vi "Drive Straight.vi"(0 "Distance (ft)":dbl) -> ()   [LabVIEW 2015]
uses:
  <vilib>/Rock Robotics/WPI/Utilities/WPI_GetSetVariantRefNum.vi
  <vilib>/Rock Robotics/WPI/RobotDrive/WPI_RobotDriveArcadeDrive_Standard(NoSaturation).vi
  navX Library v2/navX Library v2.lvlib
panel:
  in  "Ticks/Foot":dbl=442.8
  in  "Drive Straight P":dbl=0.1
  in  "Drive Straight Min":dbl=0.25
  in  "Drive Straight Max":dbl=0.75
  in  "Drive Straight Speed":dbl=0.5 format="%#_13g"
  in  "Drive Straight Tolerance":dbl=1.0
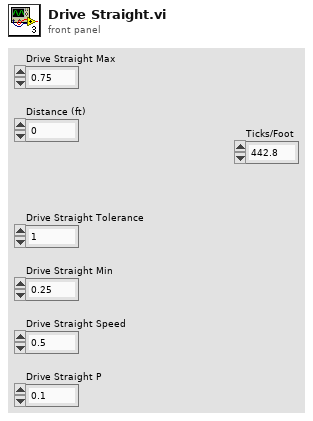
[diagram p1: front panel]
types:
  T1 = typedef "WPI_EncoderDevRef.ctl" = cluster{"DevStatus":errorcluster, "EncoderIndex":T2, "CounterIndex":T3, "DistancePerCount":dbl, "Decoding Type":T4}
  T2 = typedef "FPGA_EncoderIdx.ctl" = enum8{"Enc 0", "Enc 1", "Enc 2", "Enc 3", "Enc 4", "Enc 5", "Enc 6", "Enc 7", "Invalid"}
  T3 = typedef "FPGA_CounterCtrSystemIndex.ctl" = enum8{"Ctr 0", "Ctr 1", "Ctr 2", "Ctr 3", "Ctr 4", "Ctr 5", "Ctr 6", "Ctr 7", "Invalid"}
  T4 = typedef "WPI_EncoderType.ctl" = enum16{"1x", "2x", "4x"}
  T5 = typedef "navX Library v2.lvlib/Z900_navX_DeviceTypeDef.ctl" = cluster{"Interface":cluster{"Protocol":T6, "Update Rate (4Hz-60Hz)":u8, "navX Open TypeDef":variant}, "Notify Packet":refnum<notifier>, "Loop VI Refnum":refnum<vi>, "Ready to Close Occurrence Refnum":refnum<k4>}
  T6 = typedef "navX Library v2.lvlib/Z900_navX_ProtocolTypeDef.ctl" = enum16{"SERIAL", "I2C", "SPI"}
  T7 = cluster{"Yaw":dbl, "Roll":dbl, "Pitch":dbl, "Heading":dbl, "Fused Heading":dbl}
  T8 = typedef "WPI_RobotDriveDevRef.ctl" = cluster{"DevStatus":errorcluster, "Motors[]":T9[], "Square Inputs":bool, "Max Output":dbl}
  T9 = typedef "WPI_MotorControlDeviceRef.ctl" = cluster{"DeviceStatus":errorcluster, "Type":T10, "PWM":cluster{"PWM Channel":T11, "DeadBand":T12}, "CAN":cluster{"Device Number":u8, "Control Mode":T13, "Semaphore":T14, "Max Vout":dbl, "TalonSRX Control Mode":T15}, "Invert":bool}
  T10 = typedef "WPI_MotorControlType.ctl" = enum16{"PWM", "CAN", "CANTalonSRX"}
  T11 = typedef "FPGA_DIOPWMChannel.ctl" = enum8{"PWM 0", "PWM 1", "PWM 2", "PWM 3", "PWM 4", "PWM 5", "PWM 6", "PWM 7", "PWM 8", "PWM 9", "PWM MXP 0", "PWM MXP 1", "PWM MXP 2", "PWM MXP 3", "PWM MXP 4", "PWM MXP 5", "PWM MXP 6", "PWM MXP 7", "PWM MXP 8", "PWM MXP 9", "Invalid"}
  T12 = typedef "WPI_PWMDeadband.ctl" = cluster{"Name":string, "maxPositivePwm":i32, "minPositivePwm":i32, "centerPwm":i32, "maxNegativePwm":i32, "minNegativePwm":i32, "angularRange":u16}
  T13 = typedef "WPI_CANJaguar_ControlMode.ctl" = enum8{"Percent VBus", "Current", "Speed", "Position", "Voltage"}
  T14 = typedef "Semaphore RefNum" = refnum<k1>
  T15 = typedef "WPI_CANTalonSRX_APIControlMode.ctl" = enum8{"Percent VBus", "Speed", "Position", "Slave", "Unchanged / Invalid", "Voltage Compensation", "Current", "Motion Profile"}
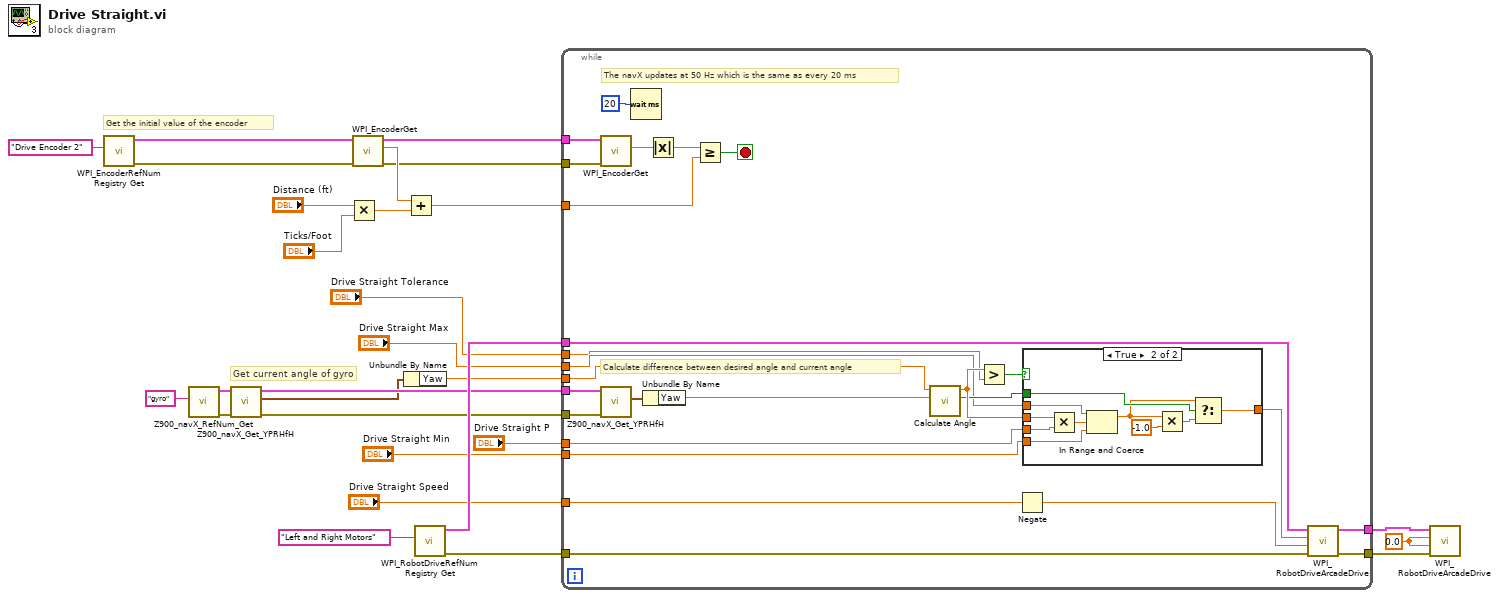
[diagram p0: block diagram]
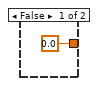
[diagram p2: hidden frame]
diagram:
  w5 = 0.0 ("Y axis value")
  # "Get the initial value of the encoder"
  # "Get current angle of gyro"
  n1 = call <vilib>:"WPI_EncoderRefNum Registry Get.vi"("refnum name"="Drive Encoder 2") -> ("error out"=w12:errorcluster, "EncoderDevRef"=w13:T1)  [unwired: 9 in]
  n2 = call "Z900_navX_RefNum_Get.vi"("refnum name"="gyro") -> ("error out"=w1:errorcluster, "navX Device"=w24:T5)  [unwired: 9 in]
  n3 = call "Z900_navX_Get_YPRHfH.vi"("error in (no error)"=w1, "navX Device"=w24) -> ("error out"=w2:errorcluster, "YRPHfH"=w23:T7, "navX Device"=w26:T5)  [unwired: 6 in, 1 out]
  n4 = Multiply(x="Distance (ft)", y="Ticks/Foot") -> (x*y=w11:dbl)
  n5 = call <vilib>:"WPI_EncoderGet.vi"("error in (no error)"=w12, "EncoderDevRef"=w13) -> ("error out"=w7:errorcluster, "Distance"=w10:dbl, "EncoderDevRef"=w8:T1)  [unwired: 4 in, 3 out]
  n6 = Unbundle By Name(w23) -> ("Yaw"=w25:dbl)
  n7 = Add(x=w10, y=w11) -> (x+y=w9:dbl)
  n8 = call <vilib>:"WPI_RobotDriveRefNum Registry Get.vi"("refnum name"="Left and Right Motors") -> ("error out"=w3:errorcluster, "RobotDriveDevRef"=w28:T8)  [unwired: 1 in, 8 out]
  n9 = while {
    tunnel: w25 -> [w54]
    tunnel: w26 -> [w53]
    tunnel: w28 -> [w52]
    tunnel: "Drive Straight P" -> [w41]
    tunnel: "Drive Straight Min" -> [w40]
    tunnel: "Drive Straight Max" -> [w39]
    tunnel: "Drive Straight Tolerance" -> [w38]
    tunnel: "Drive Straight Speed" -> [w37]
    tunnel: w9 -> [w36]
    tunnel: w8 -> [w35]
    tunnel: w7 -> [w34]
    tunnel: [w32] -> w6
    tunnel: [w31] -> w4
    tunnel: w3 -> [w30]
    tunnel: w2 -> [w29]
    stop <- w51 stop-if-true
    # "The navX updates at 50 Hz which is the same as every 20 ms"
    # "Calculate difference between desired angle and current angle"
    n10 = call <vilib>:"WPI_EncoderGet.vi"("error in (no error)"=w34, "EncoderDevRef"=w35) -> ("Distance"=w33:dbl)  [unwired: 4 in, 5 out]
    n11 = call "Z900_navX_Get_YPRHfH.vi"("error in (no error)"=w29, "navX Device"=w53) -> ("YRPHfH"=w50:T7)  [unwired: 6 in, 3 out]
    n12 = Wait (ms)(milliseconds to wait=u32 20) -> ()  [unwired: 1 out]
    n13 = Unbundle By Name(w50) -> ("Yaw"=w49:dbl)
    n14 = Absolute Value(x=w33) -> (abs(x)=w42:dbl)
    n15 = Greater Or Equal?(x=w42, y=w36) -> (x >= y?=w51:bool)
    n16 = call "Calculate Angle.vi"("Current Angle"=w49, "Target Angle"=w54) -> ("Clockwise"=w45:bool, "Delta Angle"=w46:dbl)  [unwired: 8 in]
    n17 = Greater?(x=w46, y=w38) -> (0:w47:bool)
    n18 = Negate(x=w37) -> (-x=w43:dbl)
    n19 = case shown="True" w47 {
      tunnel: [0.0 w62] -> w48
      tunnel: w46 -> [_ w65]
      tunnel: w45 -> [_ w63]
      tunnel: w41 -> [_ w58]
      tunnel: w40 -> [_ w57]
      tunnel: w39 -> [_ w56]
      frame False {
      }
      frame True {
        n20 = Multiply(x=w65, y=w58) -> (x*y=w64:dbl)
        n21 = In Range and Coerce(upper limit=w56, x=w64, lower limit=w57) -> (coerced(x)=w59:dbl)  [unwired: 1 out]
        n22 = Multiply(x=w59, y=-1.0) -> (x*y=w60:dbl)
        n23 = Select(t=w59, s=w63, f=w60) -> (s? t:f=w62:dbl)
      }
    }
    n24 = call-poly <vilib>:"WPI_RobotDriveArcadeDrive.vi"("error in (no error)"=w30, "Y axis value"=w43, "X axis value"=w48, "RobotDriveDevRef"=w52) -> ("error out"=w31:errorcluster, "RobotDriveDevRef"=w32:T8)  [unwired: 6 out]
  }
  n25 = call-poly <vilib>:"WPI_RobotDriveArcadeDrive.vi"("error in (no error)"=w4, "Y axis value"=w5, "X axis value"=w5, "RobotDriveDevRef"=w6) -> ()  [unwired: 8 out]
